vi "autoMotionProfileGenerate.vi"(6 "T2 (s)":dbl, 8 "T1 (s)":dbl, 9 "itp (s)":dbl, 10 "Distance (ft)":dbl, 11 "Vprog (ft/s)":dbl) -> (3 "Speed steps (ft/s)":dbl[](array[numeric]))   [LabVIEW 2012]
panel:
  out "Acceleration steps (ft/s^2)":dbl[](array[numeric])
  out "Array of Computational Values":dbl[][](array[numeric])
  out "Array 2":dbl[](array[numeric])
  out "# of F2 Terms":dbl
  out "Total # of Steps":dbl
  out "# of F1 Terms":dbl
  out "N (# of steps)":dbl
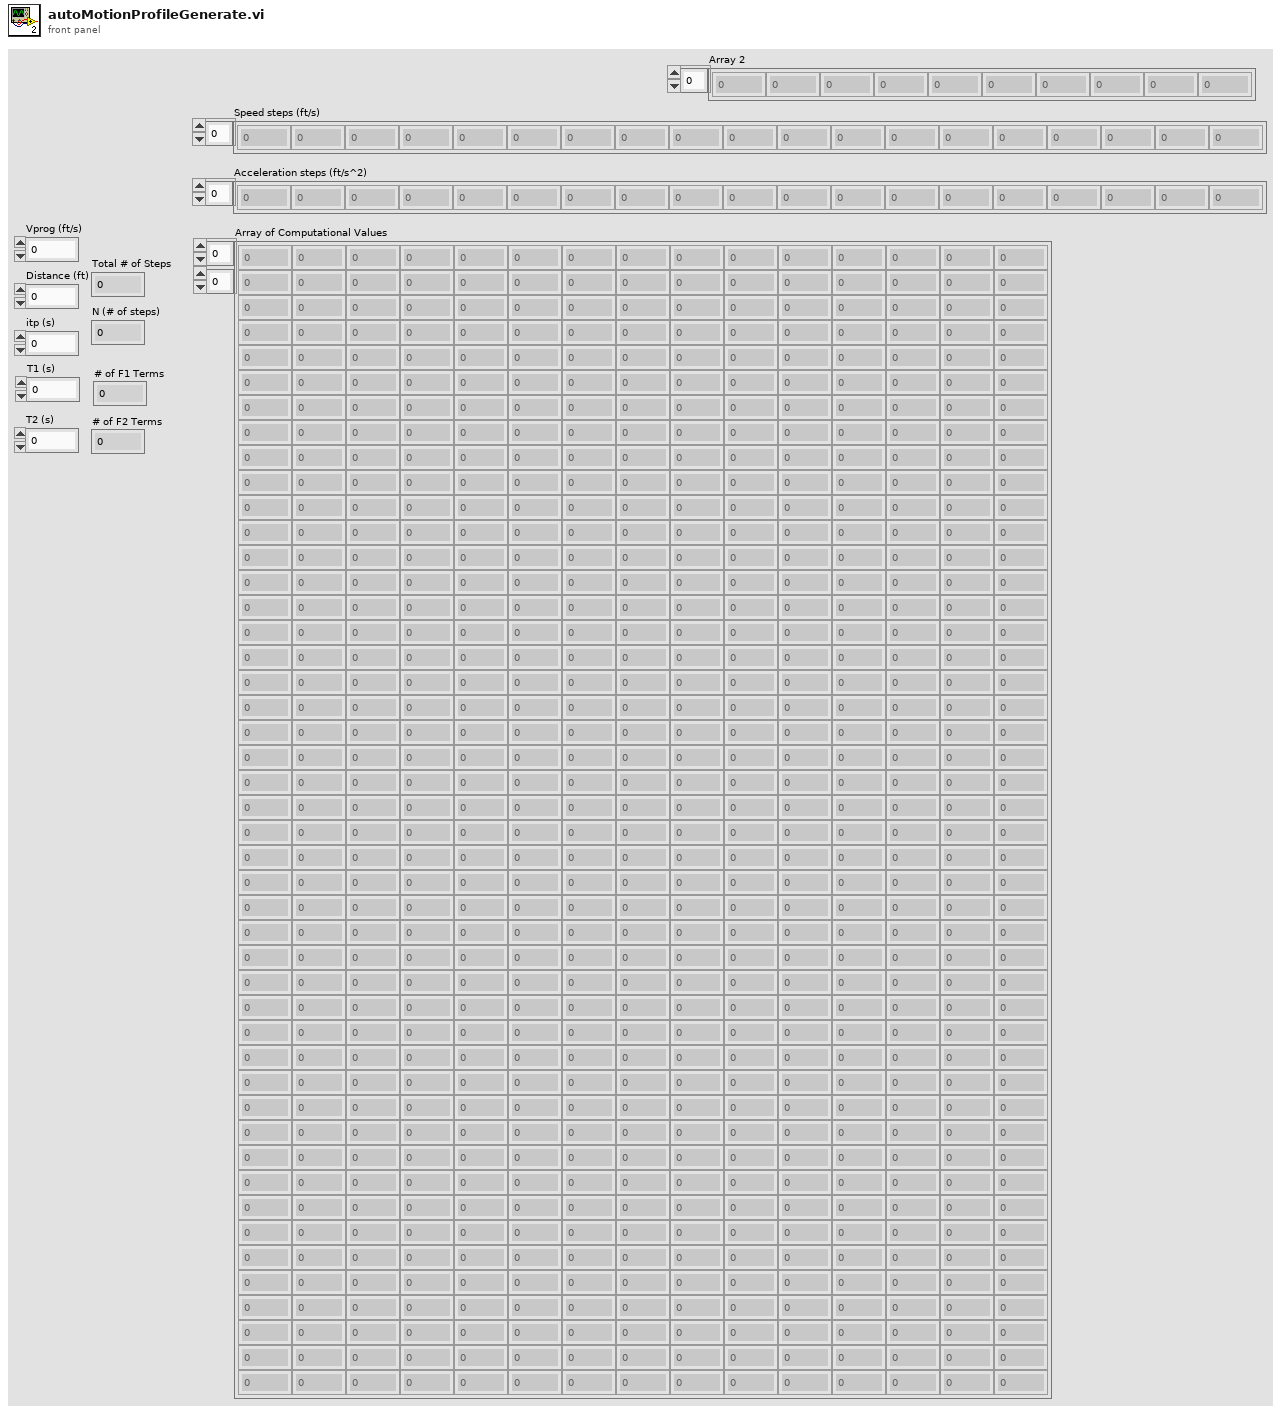
[diagram p1: front panel]
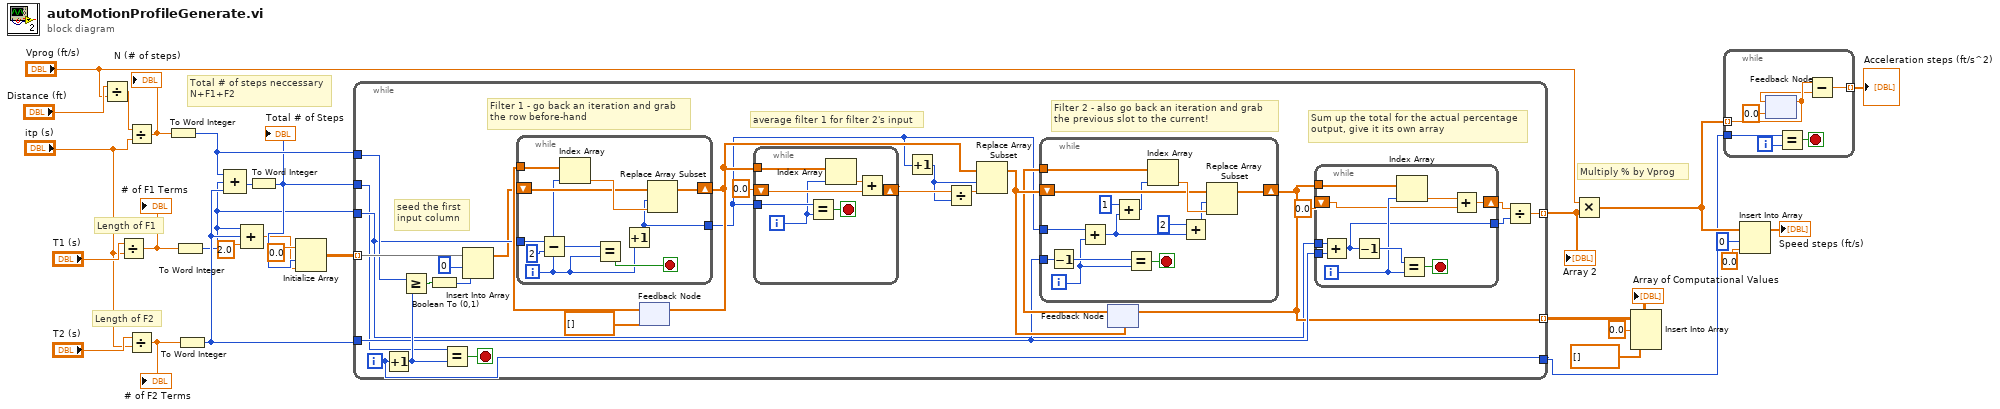
[diagram p0: block diagram]
diagram:
  # "Multiply % by Vprog"
  # "Total # of steps neccessary\nN+F1+F2"
  # "Length of F2"
  # "Length of F1"
  n1 = Divide(x="Distance (ft)", y="Vprog (ft/s)") -> (x/y=w28:dbl)
  n2 = Divide(x="T1 (s)", y="itp (s)") -> (x/y=w15:dbl)
  "# of F1 Terms" <- w15
  n3 = Divide(x=w28, y="itp (s)") -> (x/y=w18:dbl)
  "N (# of steps)" <- w18
  n4 = Divide(x="T2 (s)", y="itp (s)") -> (x/y=w14:dbl)
  "# of F2 Terms" <- w14
  n5 = To Word Integer(number=w18) -> (16bit integer=w17:i16)
  n6 = To Word Integer(number=w15) -> (16bit integer=w6:i16)
  n7 = To Word Integer(number=w14) -> (16bit integer=w16:i16)
  n8 = Compound Arithmetic op=ADD(w17, w6, w16) -> (w20:i16)
  n9 = Compound Arithmetic op=unknown(w6, w16, 2.0 ("value")) -> (w12:dbl)
  n10 = To Word Integer(number=w20) -> (16bit integer=w13:i16)
  "Total # of Steps" <- w13
  n11 = Initialize Array(0.0, w13, w12) -> (w11:dbl[][])
  n12 = while {
    tunnel: w6 -> [w34]
    tunnel: w17 -> [w54]
    tunnel: w16 -> [w40]
    tunnel: w11 -> [w56] mode=indexing
    tunnel: [w39] -> w24 mode=indexing
    tunnel: w13 -> [w33]
    tunnel: [w36] -> w2 mode=indexing
    tunnel: [w30] -> w1
    i -> [w30]
    stop <- w55 stop-if-true
    # "Sum up the total for the actual percentage output, give it its own array"
    # "Filter 2 - also go back an iteration and grab\nthe previous slot to the current!"
    # "average filter 1 for filter 2's input"
    # "seed the first \ninput column"
    # "Filter 1 - go back an iteration and grab\nthe row before-hand"
    n13 = Increment(x=w30) -> (x+1=w53:i32)
    n14 = Greater Or Equal?(x=w54, y=w53) -> (x >= y?=w51:bool)
    n15 = Boolean To (0,1)(Boolean=w51) -> (0, 1=w52:i16)
    n16 = Equal?(x=w33, y=w53) -> (x = y?=w55:bool)
    n17 = Insert Into Array(array=w56, index=0, new element=w52) -> (w32:dbl[])
    n18 = feedback #1(dbl[] []) -> (w49:dbl[])
    n19 = while {
      shift-right: [w95] -> w48
      shift-left: w32 -> [w93]
      tunnel: w49 -> [w94]
      tunnel: w34 -> [w91]
      tunnel: [w92] -> w42
      i -> [w88]
      stop <- w97 stop-if-true
      n20 = Subtract(x=w91, y=i16 2) -> (x-y=w89:i16)
      n21 = Index Array(array=w94, index=w88) -> (element=w96:dbl)
      n22 = Equal?(x=w89, y=w88) -> (x = y?=w97:bool)
      n23 = Increment(x=w88) -> (x+1=w92:i32)
      n24 = Replace Array Subset(array=w93, new element=w96, index=w92) -> (w95:dbl[])
    }
    n25 = feedback-in #1(w48) -> ()
    n26 = while {
      tunnel: w42 -> [w82]
      tunnel: w48 -> [w83]
      shift-right: [w85] -> w47
      shift-left: 0.0 -> [w84]
      i -> [w81]
      stop <- w87 stop-if-true
      n27 = Equal?(x=w82, y=w81) -> (x = y?=w87:bool)
      n28 = Index Array(array=w83, index=w81) -> (element=w86:dbl)
      n29 = Add(x=w86, y=w84) -> (x+y=w85:dbl)
    }
    n30 = Increment(x=w42) -> (x+1=w41:i32)
    n31 = Divide(x=w47, y=w41) -> (x/y=w43:dbl)
    n32 = Replace Array Subset(array=w48, new element=w43, index=w41) -> (w45:dbl[])
    n33 = feedback #2(w45) -> (w44:dbl[])
    n34 = while {
      shift-right: [w79] -> w39
      shift-left: w45 -> [w77]
      tunnel: w44 -> [w78]
      tunnel: w42 -> [w70]
      tunnel: w40 -> [w68]
      i -> [w69]
      stop <- w72 stop-if-true
      n35 = Decrement(x=w68) -> (x-1=w71:i16)
      n36 = Add(x=w70, y=w69) -> (x+y=w67:i32)
      n37 = Add(x=i16 1, y=w67) -> (x+y=w75:i32)
      n38 = Equal?(x=w71, y=w69) -> (x = y?=w72:bool)
      n39 = Index Array(array=w78, index=w75) -> (element=w80:dbl)
      n40 = Add(x=i16 2, y=w67) -> (x+y=w73:i32)
      n41 = Replace Array Subset(array=w77, new element=w80, index=w73) -> (w79:dbl[])
    }
    n42 = feedback-in #2(w39) -> ()
    n43 = while {
      tunnel: w40 -> [w64]
      tunnel: w34 -> [w63]
      tunnel: w39 -> [w62]
      shift-right: [w59] -> w37
      shift-left: 0.0 -> [w58]
      tunnel: [w57] -> w38
      i -> [w61]
      stop <- w66 stop-if-true
      n44 = Add(x=w63, y=w64) -> (x+y=w57:i16)
      n45 = Decrement(x=w57) -> (x-1=w65:i16)
      n46 = Index Array(array=w62, index=w61) -> (element=w60:dbl)
      n47 = Equal?(x=w65, y=w61) -> (x = y?=w66:bool)
      n48 = Add(x=w60, y=w58) -> (x+y=w59:dbl)
    }
    n49 = Divide(x=w37, y=w38) -> (x/y=w36:dbl)
  }
  "Array 2" <- w2
  n50 = Multiply(x="Vprog (ft/s)", y=w2) -> (x*y=w4:dbl[])
  n51 = Insert Into Array(array=w24, index (row)=0.0, new element=dbl[] []) -> (→"Array of Computational Values":dbl[][])  [unwired: 1 in]
  n52 = while {
    tunnel: w1 -> [w104]
    tunnel: w4 -> [w101] mode=indexing
    tunnel: [w98] -> w3 mode=indexing
    i -> [w103]
    stop <- w102 stop-if-true
    n53 = feedback-in #3(w101) -> ()
    n54 = feedback #3(0.0) -> (w100:dbl)
    n55 = Equal?(x=w104, y=w103) -> (x = y?=w102:bool)
    n56 = Subtract(x=w101, y=w100) -> (x-y=w98:dbl)
  }
  "Acceleration steps (ft/s^2)" <- w3
  n57 = Insert Into Array(array=w4, index=0, new element=0.0 ("new element/subarray")) -> (→"Speed steps (ft/s)":dbl[])
